vi "GetPoint.vi"(8 "error in (no error)":errorcluster, 11 "UMLClass in":refnum<class "UMLClass.lvclass">) -> (0 "error out":errorcluster, 2 "Point":refnum<class "Point.lvclass">, 3 "UMLClass out":refnum<class "UMLClass.lvclass">)   [LabVIEW 2021, in "Picture2D.lvlib" / "UMLClass.lvclass"]
uses:
  UMLClass.lvclass
  Shape/Shape.lvclass
  Point/Point.lvclass
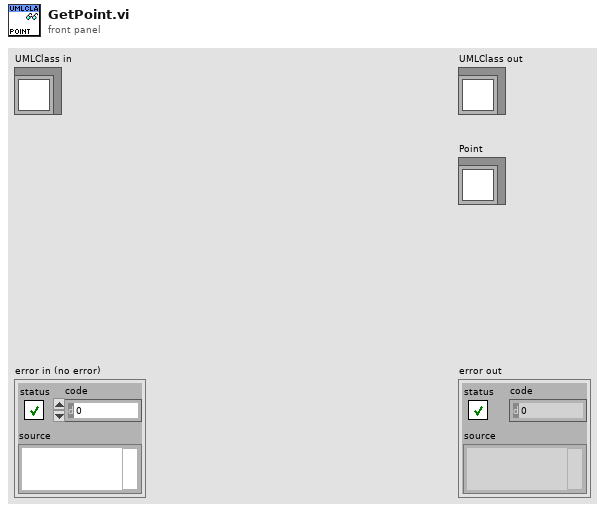
[diagram p1: front panel]
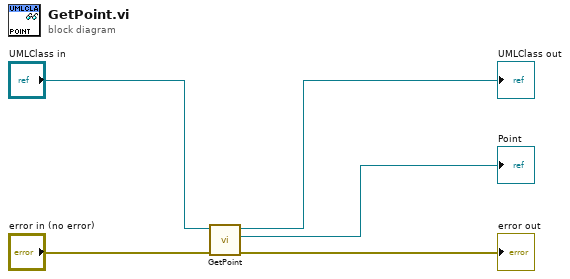
[diagram p0: block diagram]
diagram:
  n1 = call-parent "GetPoint.vi"("error in (no error)"="error in (no error)", "Picture2D in"="UMLClass in") -> ("error out"=→"error out":errorcluster, "Point"=→"Point":refnum<class "Point.lvclass">, "Picture2D out"=→"UMLClass out":refnum<class "UMLClass.lvclass">)  [unwired: 7 in]
